vi "Configure Signal (Level).vi"(0 "niUsrpRio Session":T1={"FPGA Interface"=refnum, "RIO Interface Number"=0, "Data Clock Rate"=0, "FPGA Data Clock Rate"=0, "Global Settings Register Bus"=refnum, "Radio 0 Settings Register Bus"=refnum, "Radio 1 Settings Register Bus"=refnum, "Radio Settings Bus Semaphore"=refnum, "DB Queues"=[], "Characterization Data Valid?"=FALSE, "EEPROM Header"={"Checksum"=0, "Product Code"=0, "Hardware Current Version"=0, "Hardware Oldest Compatible Version"=0, "EEPROM Map Current Version"=0, "EEPROM Map Oldest Compatible Version"=0, "User Password"="", "Pointer to Factory Header"=0, "Pointer to User Header"=0, "Recommended Interval"=0, "Number of Reserved Bytes"=9, "Number of Daughterboards"=0, "Daughterboard IDs"=[], "Daughterboard Serial Numbers"=[]}, "Device Data Header"={"Checksum"=0, "Number of Channels"=0, "Number of Gain Settings"=[], "Pointer to Characterization Data"=[], "Number of Reserved Bytes"=27, "Number of Frequencies"=[]}, "EEPROM Characterization Header"={"Checksum"=0, "Date"=timestamp(0 s since 1904-01-01), "Temperature"=0.0, "Misc. Info"="", "Pointer to Device Data Header"=0, "Number of Reserved Bytes"=28}, "Characterization Data"=[], "FPGA Current Version"=0, "FPGA Oldest Compatible Version"=0, "Fixed Logic Current Version"=0, "Fixed Logic Oldest Compatible Version"=0, "FPGA Radio Settings Bus Current Version"=0, "FPGA Radio Settings Bus Oldest Compatible Version"=0, "FPGA Board Config Current Version"=0, "FPGA Board Config Oldest Compatible Version"=0, "Daughterboard Clock Rate"=0, "daughterboard configuration session handles"=[]} {"Daughterboard Clock Rate" format="%#.3pHz"; "FPGA Data Clock Rate" format="%#.3pHz"; "Data Clock Rate" format="%#.3pHz"; "Characterization Data"."Frequencies [Hz]" format="%#_6p"; "EEPROM Characterization Header"."Pointer to Device Data Header" format="%x"; "EEPROM Characterization Header"."Checksum" format="%x"; "Device Data Header"."Pointer to Characterization Data" format="%x"; "Device Data Header"."Checksum" format="%x"; "EEPROM Header"."Pointer to User Header" format="%x"; "EEPROM Header"."Pointer to Factory Header" format="%x"; "EEPROM Header"."Product Code" format="%x"; "EEPROM Header"."Checksum" format="%x"}, 1 "scope":string(combo)="rx", 2 "Correct Impairments?":bool=TRUE, 5 "sample rate [S/s]":dbl=10000000.0 caption="Sample Rate [S/s]" min=1.0 max=250000000.0 format="%#.3pS/s", 7 "frequency [Hz]":dbl=2450000000.0 caption="Frequency [Hz]" format="%#.3pHz", 9 "level [dBm]":dbl=-10.0 caption="Level [dBm]" format="%#_gdBm", 11 "error in":errorcluster, 12 "Active Antenna":string(combo)="RX1", 13 "LO frequency [Hz]":dbl=-1.0 caption="LO Frequency [Hz]" format="%#.3pHz") -> (3 "coerced vertical range [Vpp]":dbl caption="Coerced Vertical Range [Vpp]" format="%#.3pV", 4 "niUsrpRio Session (out)":T1={"FPGA Interface"=refnum, "RIO Interface Number"=0, "Data Clock Rate"=0, "FPGA Data Clock Rate"=0, "Global Settings Register Bus"=refnum, "Radio 0 Settings Register Bus"=refnum, "Radio 1 Settings Register Bus"=refnum, "Radio Settings Bus Semaphore"=refnum, "DB Queues"=[], "Characterization Data Valid?"=FALSE, "EEPROM Header"={"Checksum"=0, "Product Code"=0, "Hardware Current Version"=0, "Hardware Oldest Compatible Version"=0, "EEPROM Map Current Version"=0, "EEPROM Map Oldest Compatible Version"=0, "User Password"="", "Pointer to Factory Header"=0, "Pointer to User Header"=0, "Recommended Interval"=0, "Number of Reserved Bytes"=9, "Number of Daughterboards"=0, "Daughterboard IDs"=[], "Daughterboard Serial Numbers"=[]}, "Device Data Header"={"Checksum"=0, "Number of Channels"=0, "Number of Gain Settings"=[], "Pointer to Characterization Data"=[], "Number of Reserved Bytes"=27, "Number of Frequencies"=[]}, "EEPROM Characterization Header"={"Checksum"=0, "Date"=timestamp(0 s since 1904-01-01), "Temperature"=0.0, "Misc. Info"="", "Pointer to Device Data Header"=0, "Number of Reserved Bytes"=28}, "Characterization Data"=[], "FPGA Current Version"=0, "FPGA Oldest Compatible Version"=0, "Fixed Logic Current Version"=0, "Fixed Logic Oldest Compatible Version"=0, "FPGA Radio Settings Bus Current Version"=0, "FPGA Radio Settings Bus Oldest Compatible Version"=0, "FPGA Board Config Current Version"=0, "FPGA Board Config Oldest Compatible Version"=0, "Daughterboard Clock Rate"=0, "daughterboard configuration session handles"=[]} {"Daughterboard Clock Rate" format="%#.3pHz"; "FPGA Data Clock Rate" format="%#.3pHz"; "Data Clock Rate" format="%#.3pHz"; "Characterization Data"."Frequencies [Hz]" format="%#_6p"; "EEPROM Characterization Header"."Pointer to Device Data Header" format="%x"; "EEPROM Characterization Header"."Checksum" format="%x"; "Device Data Header"."Pointer to Characterization Data" format="%x"; "Device Data Header"."Checksum" format="%x"; "EEPROM Header"."Pointer to User Header" format="%x"; "EEPROM Header"."Pointer to Factory Header" format="%x"; "EEPROM Header"."Product Code" format="%x"; "EEPROM Header"."Checksum" format="%x"}, 6 "coerced sample rate [S/s]":dbl=10000000.0 caption="Coerced Sample Rate [S/s]" min=1.0 max=250000000.0 format="%#.3pS/s", 8 "coerced frequency [Hz]":dbl=2450000000.0 caption="Coerced Frequency [Hz]" format="%#.3pHz", 10 "coerced level [dBm]":dbl=-10.0 caption="Coerced Level [dBm]" format="%#_gdBm", 14 "coerced LO frequency [Hz]":dbl=-1.0 caption="coerced LO Frequency [Hz]" format="%#.3pHz", 15 "error out":errorcluster)   [LabVIEW 2021]
doc: "Configures the DSP and signal path for the channel based on the input <B>signal parameters</B>.\n\n<B>Input Parameters</B>\n\n<B>Sample Rate</B> the requested rate, in samples per second, the signal will be sampled at.\n\n<B>Frequency</B> is the requested frequency, in hertz, to acquire the signal from/generate the signal at.\n\n<B>Level</B> is the requested power level, in dBm, of the signal.\n\n<B>Gain</B> is the requested amount of gain, in dB.\n\n<B>LO Frequency</B> is the requested frequency, in hertz, to tune the local oscillator to. The default value of -1 sets the LO to the value of the 'Frequency' input. If the value is not -1, the LO will be set to that value, and the DSP will handle the difference between the 'Frequency' and the 'LO Frequency'.\n\n<B>Active Antenna</B> is the antenna to use for this channel.\n\n<B>Correct Impairments</B> applies the correction information of the device to the signal."
uses:
  <instrlib>/niUsrpRio/Config/v1/Host/Public/niUsrpRio Session.ctl
  <instrlib>/_niInstr/Register Bus/v0/Host/Public/Register Bus Session.ctl
  <instrlib>/_niInstr/Register Bus/v0/Host/Private/Session Data.ctl
  <instrlib>/niUsrpRio/Config/v1/Host/Private/DB Queue Reference.ctl
  <instrlib>/niUsrpRio/Config/v1/Host/Private/Daughterboard Data.ctl
  <instrlib>/niUsrpRio/Config/v1/Host/Private/ATR state data.ctl
  <instrlib>/niUsrpRio/Config/v1/Host/Private/Antenna Configuration.ctl
  <instrlib>/niUsrpRio/Config/v1/Host/Private/CPLD Power Mode.ctl
  <instrlib>/niUsrpRio/Config/v1/Host/Public/EEPROM Header.ctl
  <instrlib>/niUsrpRio/Config/v1/Host/Public/EEPROM Device Data Header.ctl
  <instrlib>/niUsrpRio/Config/v1/Host/Public/EEPROM Characterization Header.ctl
  <instrlib>/niUsrpRio/Config/v1/Host/Public/Characterization Data.ctl
  <instrlib>/niUsrpRio/Config/v1/Host/Public/IQ Imbalance.ctl
  Configure Signal Parameters.ctl
  Configure Signal Mode.ctl
  <instrlib>/_niInstr/Register Bus/v0/Host/niInstr Register Bus v0 Host.lvlib
  <instrlib>/niUsrpRio/Config/v1/Host/niUsrpRio Config v1 Host.lvlib
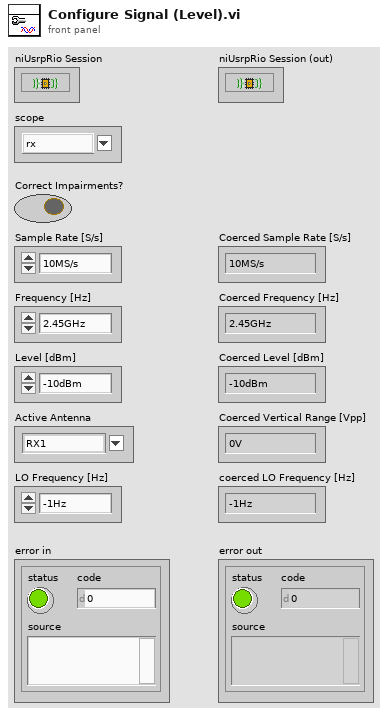
[diagram p1: front panel]
types:
  T1 = typedef "niUsrpRio Config v1 Host.lvlib/niUsrpRio Session.ctl" = cluster{"FPGA Interface":refnum<k20>, "RIO Interface Number":u32, "Data Clock Rate":u32, "FPGA Data Clock Rate":u32, "Global Settings Register Bus":T2, "Radio 0 Settings Register Bus":T2, "Radio 1 Settings Register Bus":T2, "Radio Settings Bus Semaphore":T3, "DB Queues":T4[], "Characterization Data Valid?":bool, "EEPROM Header":T5, "Device Data Header":T6, "EEPROM Characterization Header":T7, "Characterization Data":T8[], "FPGA Current Version":u32, "FPGA Oldest Compatible Version":u32, "Fixed Logic Current Version":u32, "Fixed Logic Oldest Compatible Version":u32, "FPGA Radio Settings Bus Current Version":u32, "FPGA Radio Settings Bus Oldest Compatible Version":u32, "FPGA Board Config Current Version":u32, "FPGA Board Config Oldest Compatible Version":u32, "Daughterboard Clock Rate":u32, "daughterboard configuration session handles":u64[]}
  T2 = typedef "niInstr Register Bus v0 Host.lvlib/Register Bus Session.ctl" = refnum<queue>
  T3 = typedef "Semaphore RefNum" = refnum<k1>
  T4 = typedef "niUsrpRio Config v1 Host.lvlib/DB Queue Reference.ctl" = refnum<queue>
  T5 = typedef "niUsrpRio Config v1 Host.lvlib/EEPROM Header.ctl" = cluster{"Checksum":u32, "Product Code":u16, "Hardware Current Version":u16, "Hardware Oldest Compatible Version":u16, "EEPROM Map Current Version":u16, "EEPROM Map Oldest Compatible Version":u16, "User Password":string, "Pointer to Factory Header":u32, "Pointer to User Header":u32, "Recommended Interval":u16, "Number of Reserved Bytes":i32, "Number of Daughterboards":u8, "Daughterboard IDs":u16[], "Daughterboard Serial Numbers":string[]}
  T6 = typedef "niUsrpRio Config v1 Host.lvlib/EEPROM Device Data Header.ctl" = cluster{"Checksum":u32, "Number of Channels":u8, "Number of Gain Settings":u16[], "Pointer to Characterization Data":u32[], "Number of Reserved Bytes":i32, "Number of Frequencies":u16[]}
  T7 = typedef "niUsrpRio Config v1 Host.lvlib/EEPROM Characterization Header.ctl" = cluster{"Checksum":u32, "Date":timestamp, "Temperature":sgl, "Misc. Info":string, "Pointer to Device Data Header":u32, "Number of Reserved Bytes":i32}
  T8 = typedef "niUsrpRio Config v1 Host.lvlib/Characterization Data.ctl" = cluster{"Gains[dB]":dbl[], "Frequencies [Hz]":dbl[], "IQ Imbalance Table":T9[], "Measured Gains[dB]":dbl[][]}
  T9 = typedef "niUsrpRio Config v1 Host.lvlib/IQ Imbalance.ctl" = cluster{"Gain Imbalance [linear]":dbl, "Phase Imbalance [radians]":dbl, "Offset":cdb}
  T10 = typedef "Configure Signal Mode.ctl" = enum16{"Gain", "Level"}
  T11 = typedef "Configure Signal Parameters.ctl" = cluster{"gain/level":dbl, "sample rate [S/s]":dbl, "frequency [Hz]":dbl, "LO frequency [Hz]":dbl, "active antenna":string}
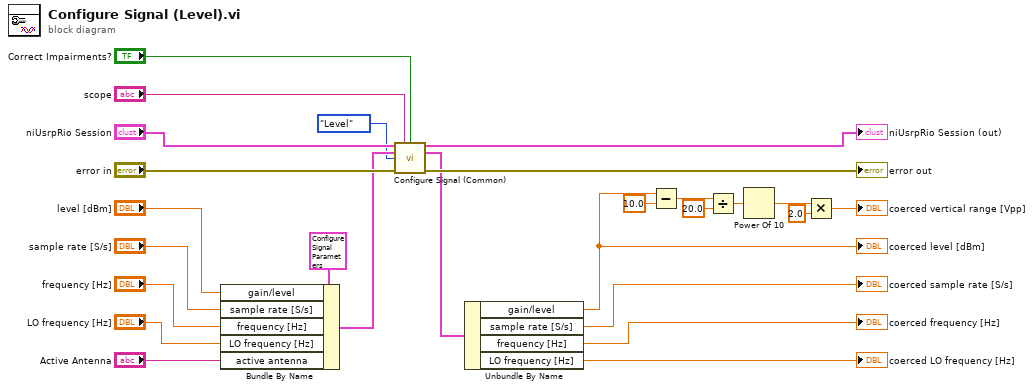
[diagram p0: block diagram]
diagram:
  n1 = Bundle By Name(cluster=T11 {"gain/level"=0.0, "sample rate [S/s]"=10000000.0, "frequency [Hz]"=2450000000.0, "LO frequency [Hz]"=-1.0, "active antenna"="RX1"} ("signal parameters"), "gain/level"="level [dBm]", "sample rate [S/s]"="sample rate [S/s]", "frequency [Hz]"="frequency [Hz]", "LO frequency [Hz]"="LO frequency [Hz]", "active antenna"="Active Antenna") -> (w23:T11)
  n2 = call "Configure Signal (Common).vi"("niUsrpRio Session"="niUsrpRio Session", "scope"="scope", "Correct Impairments?"="Correct Impairments?", "signal parameters"=w23, "Configure Signal Mode"=Configure_Signal_Mode."Level", "error in"="error in") -> ("niUsrpRio Session (out)"=→"niUsrpRio Session (out)":T1, "coerced signal parameters"=w22:T11, "error out"=→"error out":errorcluster)  [unwired: 7 in]
  n3 = Unbundle By Name(w22) -> ("gain/level"=w2:dbl, "sample rate [S/s]"=→"coerced sample rate [S/s]":dbl, "frequency [Hz]"=→"coerced frequency [Hz]":dbl, "LO frequency [Hz]"=→"coerced LO frequency [Hz]":dbl)
  "coerced level [dBm]" <- w2
  n4 = Subtract(x=w2, y=10.0) -> (x-y=w5:dbl)
  n5 = Divide(x=w5, y=20.0) -> (x/y=w4:dbl)
  n6 = Power Of 10(x=w4) -> (10^x=w3:dbl)
  n7 = Multiply(x=w3, y=2.0) -> (x*y=→"coerced vertical range [Vpp]":dbl)
